vi "Build_Read Device Identification.vi"(8 "error in (no error)":errorcluster, 9 "object ID":u8, 10 "read device ID code":T1=1 items=["Basic"=1, "Regular"=2, "Extended"=3, "Single Object"=4]) -> (0 "error out":errorcluster, 3 "MB_PDU":T2={"Function Code"=1, "Data"=[], "RTU_DataBytes"=0})   [LabVIEW 2021, in "MB Master.lvlib"]
doc: "Builds PDU for Read Device Identification (function code 43 / 14)."
uses:
  <vilib>/Plasmionique/MB Master/MB Master.lvlib
  <vilib>/Plasmionique/MB Master/MB_PDU/MB_PDU_Cluster.ctl
  <vilib>/Plasmionique/MB Master/MB_PDU/MB_ReadDevID Codes.ctl
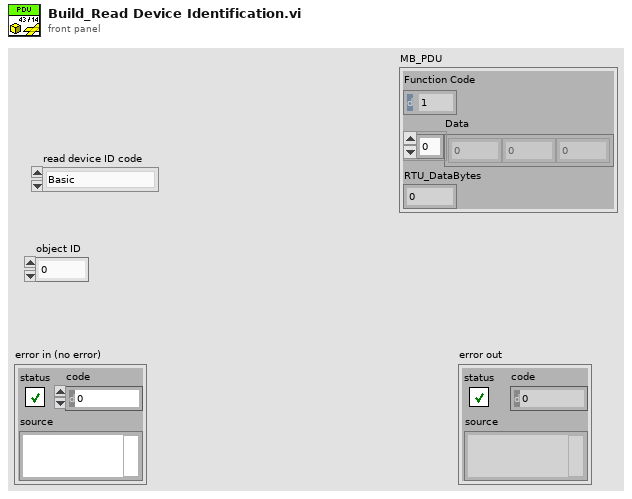
[diagram p1: front panel]
types:
  T1 = typedef "MB Master.lvlib/MB_ReadDevID Codes.ctl" = u8
  T2 = typedef "MB Master.lvlib/MB_PDU_Cluster.ctl" = cluster{"Function Code":u8, "Data":u8[], "RTU_DataBytes":i32}
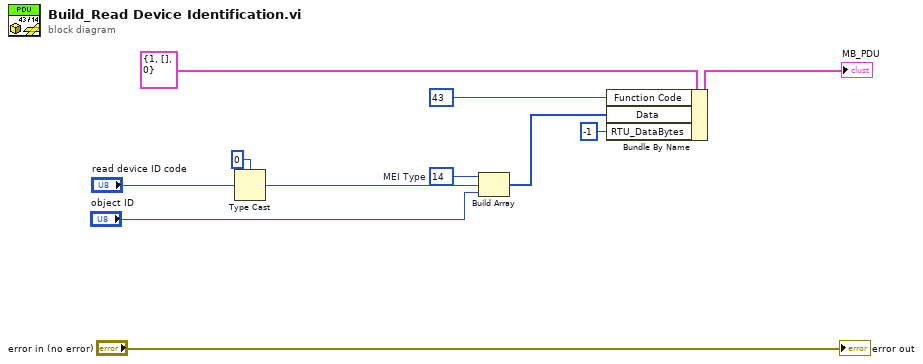
[diagram p0: block diagram]
diagram:
  w5 = u8 14  # MEI Type
  n1 = Type Cast(type=u8 0, x="read device ID code") -> (*(type *) &x=w2:u8)
  n2 = Build Array(w5, w2, "object ID") -> (w7:u8[])
  n3 = Bundle By Name(cluster=T2 {"Function Code"=1, "Data"=[], "RTU_DataBytes"=0} ("Modbus Serial New.lvlib:MB_PDU.lvclass"), "Function Code"=u8 43, "Data"=w7, "RTU_DataBytes"=-1) -> (→"MB_PDU":T2)
  "error out" <- "error in (no error)"
